vi "CLD 5 Parse Config Data File.vi"(8 "error in (no error)":errorcluster, 10 "Array In":T1[][](array[typedef])=[[{"Numeric"=1.25, "Boolean"=FALSE, "String"="One"}, {"Numeric"=1.35, "Boolean"=TRUE, "String"="Two"}, {"Numeric"=1.5, "Boolean"=FALSE, "String"="Three"}, {"Numeric"=1.0, "Boolean"=TRUE, "String"="Four"}], [{"Numeric"=2.0, "Boolean"=TRUE, "String"="Five"}, {"Numeric"=0.75, "Boolean"=FALSE, "String"="Six"}, {"Numeric"=0.9, "Boolean"=TRUE, "String"="Seven"}, {"Numeric"=0.75, "Boolean"=FALSE, "String"="Eight"}]], 11 "Get/Set":enum16{"Get", "Set"}(ring)) -> (0 "error out":errorcluster, 3 "Array Out":T1[][](array[typedef]))   [LabVIEW 2015]
doc: "CLD 5 exercise"
uses:
  CLD 5 Data Cluster.ctl
panel:
  out "String":string
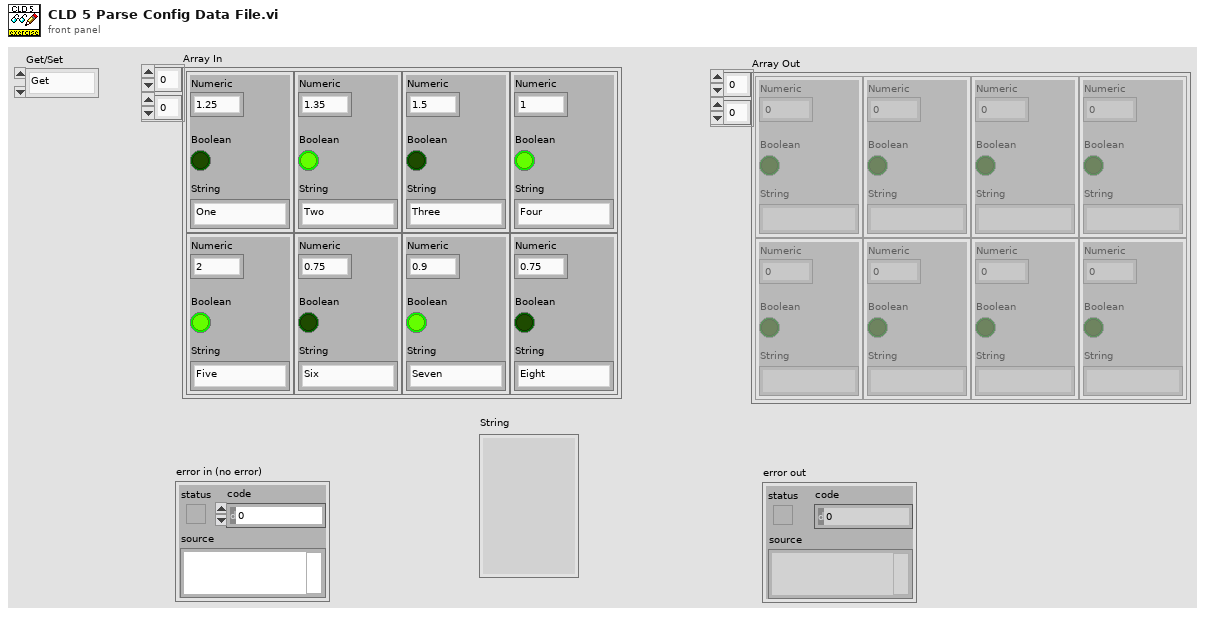
[diagram p1: front panel]
types:
  T1 = typedef "CLD 5 Data Cluster.ctl" = cluster{"Numeric":dbl, "Boolean":bool, "String":string}
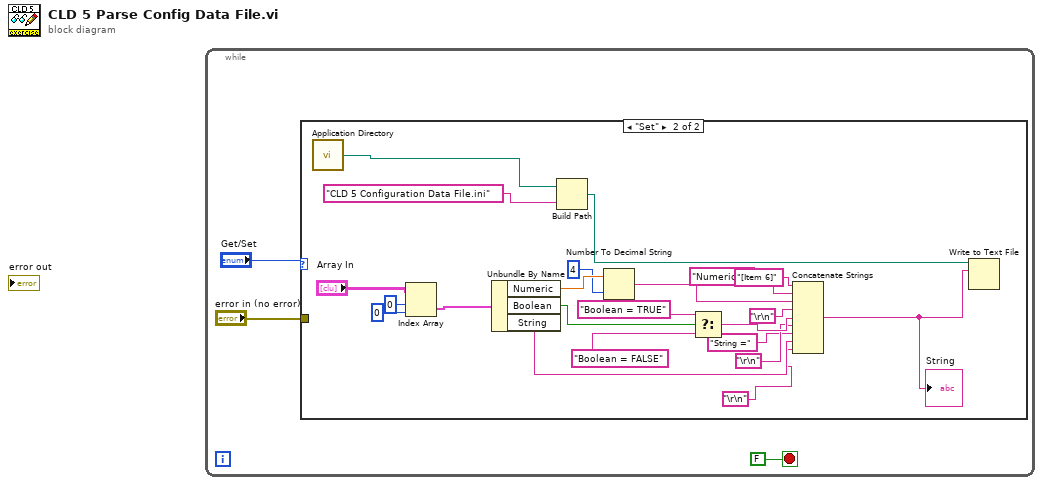
[diagram p0: block diagram]
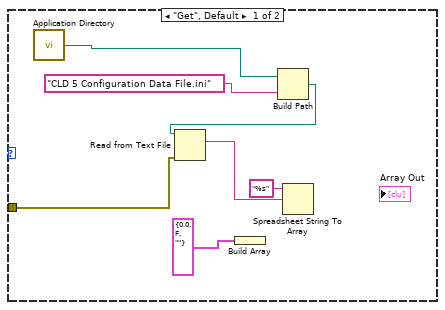
[diagram p2: hidden frame]
diagram:
  n1 = while {
    stop <- FALSE stop-if-true
    n2 = case shown="\"Set\"" "Get/Set" {
      tunnel: "error in (no error)" -> [w8 _]
      frame "Get", Default {
        n3 = call <vilib>:"Application Directory.vi"() -> ("Application Directory"=w5:path)
        n4 = Build Array(T1 {"Numeric"=0.0, "Boolean"=FALSE, "String"=""} ("Cluster")) -> ()  [unwired: 1 out]
        n5 = Build Path(base path=w5, name or relative path="CLD 5 Configuration Data File.ini") -> (appended path=w9:path)
        n6 = Read from Text File(file (use dialog)=w9, error in=w8) -> (text=w7:string)  [unwired: 1 in, 4 out]
        n7 = Spreadsheet String To Array(format string="%s", spreadsheet string=w7) -> ()  [unwired: 2 in, 1 out]
      }
      frame "Set" {
        n8 = call <vilib>:"Application Directory.vi"() -> ("Application Directory"=w31:path)
        n9 = Index Array(array="Array In", index (row)=0, index (col)=0 ("disabled index (col)")) -> (element=w26:T1)
        n10 = Unbundle By Name(w26) -> ("Numeric"=w25:dbl, "Boolean"=w23:bool, "String"=w14:string)
        n11 = Build Path(base path=w31, name or relative path="CLD 5 Configuration Data File.ini") -> (appended path=w30:path)
        n12 = Number To Decimal String(number=w25, width (-)=i16 4) -> (decimal integer string=w19:string)
        n13 = Select(t="Boolean = TRUE", s=w23, f="Boolean = FALSE") -> (s? t:f=w17:string)
        n14 = Concatenate Strings("[Item 6]" ("string"), "Numeric =" ("string"), w19, "\r\n", w17, "\r\n", "String =" ("string"), w14, "\r\n") -> (w11:string)
        "String" <- w11
        n15 = Write to Text File(file (use dialog)=w30, text=w11) -> ()  [unwired: 2 in, 3 out]
      }
    }
  }
